vi "Launch Asynchronous Execution Units.vi"(8 "error in (no error)":errorcluster, 10 "RTStateVariables in":T2 {"Inline Execution Units"."Outgoing Data References"."Data Reference" format="%.0x"; "Inline Execution Units"."Incoming Data References" format="%.0x"}, 11 "Device Ref in":T1 format="%.0x") -> (0 "error out":errorcluster, 2 "RTStateVariables out":T2 {"Inline Execution Units"."Outgoing Data References"."Data Reference" format="%.0x"; "Inline Execution Units"."Incoming Data References" format="%.0x"}, 3 "Device Ref out":T1 format="%.0x")   [LabVIEW 2020, in "Communication Bus Template Engine.lvlib" / "Custom Device.lvlib"]
uses:
  Custom Device.lvlib
  RTStateVariables.ctl
  <vilib>/NI/NIVS Inline Async API/_VS Inline Async API/VS Inline Async API/VS Inline Async API.lvclass
  Inline Execution Unit Runtime Information.ctl
  Interfaces/Execution Unit/Execution Unit.lvclass
  <vilib>/NI VeriStand/Custom Device API/Data Reference.ctl
  <vilib>/NI VeriStand/Custom Device API/Block Data Reference.ctl
  Asynchronous Execution Unit Runtime Information.ctl
  <vilib>/NI VeriStand/Custom Device API/Custom Device Item Ref.ctl
  <vilib>/NI VeriStand/Custom Device API/Custom Device API.lvlib
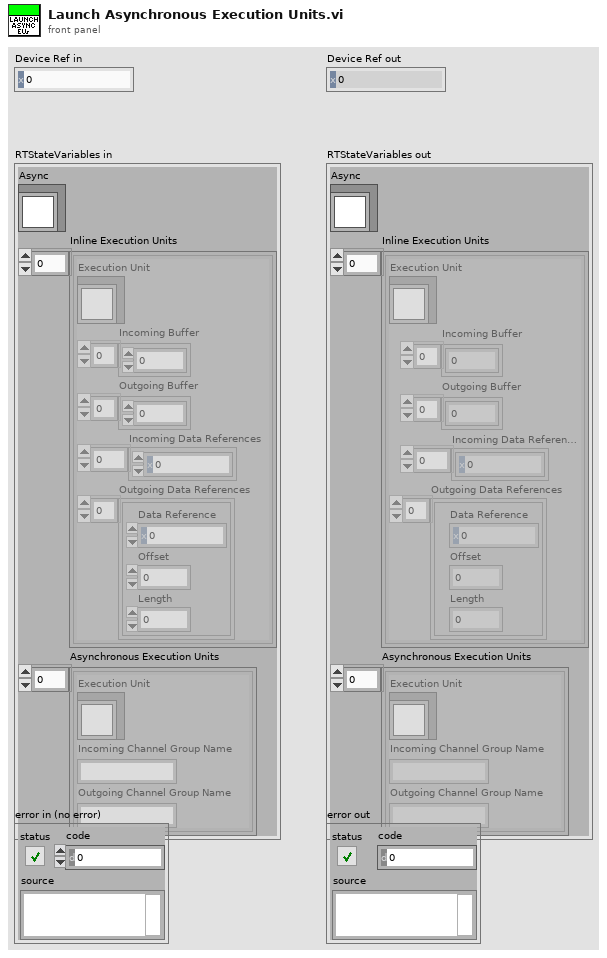
[diagram p1: front panel]
types:
  T1 = typedef "Custom Device API.lvlib/Custom Device Item Ref.ctl" = u64
  T2 = typedef "Communication Bus Template Engine.lvlib/Custom Device.lvlib/RTStateVariables.ctl" = cluster{"Async":refnum<class "VS Inline Async API.lvclass">, "Inline Execution Units":T3[], "Asynchronous Execution Units":T6[]}
  T3 = typedef "Communication Bus Template Engine.lvlib/Custom Device.lvlib/Inline Execution Unit Runtime Information.ctl" = cluster{"Execution Unit":refnum<class "Execution Unit.lvclass">, "Incoming Buffer":dbl[], "Outgoing Buffer":dbl[], "Incoming Data References":T4[], "Outgoing Data References":T5[]}
  T4 = typedef "Custom Device API.lvlib/Data Reference.ctl" = i32
  T5 = typedef "Custom Device API.lvlib/Block Data Reference.ctl" = cluster{"Data Reference":T4, "Offset":u64, "Length":u64}
  T6 = typedef "Communication Bus Template Engine.lvlib/Custom Device.lvlib/Asynchronous Execution Unit Runtime Information.ctl" = cluster{"Execution Unit":refnum<class "Execution Unit.lvclass">, "Incoming Channel Group Name":string, "Outgoing Channel Group Name":string}
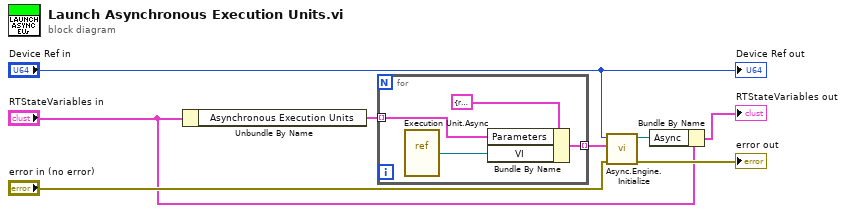
[diagram p0: block diagram]
diagram:
  n1 = Unbundle By Name("RTStateVariables in") -> ("Asynchronous Execution Units"=w2:T6[])
  n2 = for {
    tunnel: w2 -> [w9] mode=indexing
    tunnel: [w11] -> w1 mode=indexing
    n3 = vi-ref "Execution Unit.Async.vi"() -> (w10:refnum<vi>)
    n4 = Bundle By Name(cluster=cluster{"VI":refnum<vi>, "Parameters":variant} {"VI"=refnum, "Parameters"=variant} ("Process"), "Parameters"=w9, "VI"=w10) -> (w11:cluster{"VI":refnum<vi>, "Parameters":variant})
  }
  n5 = call <vilib>:"Async.Engine.Initialize.vi"("error in (no error)"="error in (no error)", "Processes"=w1, "Custom Device Ref"="Device Ref in") -> ("error out"=→"error out":errorcluster, "Async"=w4:refnum<class "VS Inline Async API.lvclass">)  [unwired: 7 in]
  n6 = Bundle By Name(cluster="RTStateVariables in", "Async"=w4) -> (→"RTStateVariables out":T2)
  "Device Ref out" <- "Device Ref in"
